vi "Status Created Events.vi"(7 "jettl in":refnum<class "jettl.lvclass">, 10 "Queue Mailbox":refnum<data-value>) -> (0 "Created Event Count":i32, 1 "Created Event Aliases":string[](array[string]), 2 "Created Event Exist?":bool, 5 "jettl out":refnum<class "jettl.lvclass">)   [LabVIEW 2021, in "jettl.lvlib" / "Addresses.lvlib"]
uses:
  Addresses.lvlib
  Addresses/Addresses.lvclass
  jettl/jettl.lvclass
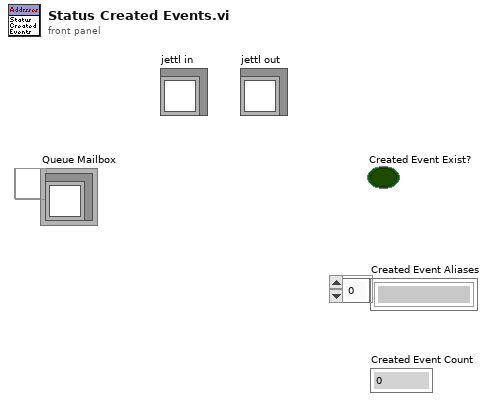
[diagram p1: front panel]
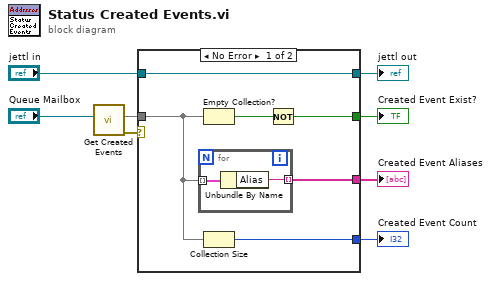
[diagram p0: block diagram]
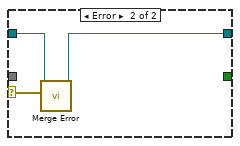
[diagram p2: hidden frame]
diagram:
  n1 = call "Get Created Events.vi"("Queue Mailbox"="Queue Mailbox") -> ("error out"=w3:errorcluster, "Created Events"=w2:map{string, refnum<data-value>})  [unwired: 9 in]
  n2 = case shown="No Error" w3 {
    selector: w3 -> [_ w17]
    tunnel: [w13 _] -> w8
    tunnel: [w12 _] -> w7
    tunnel: [w11 _] -> w6
    tunnel: w2 -> [w10 _]
    tunnel: [w9 w18] -> w5
    tunnel: "jettl in" -> [w9 w19]
    frame No Error {
      n3 = for {
        tunnel: [w15] -> w12 mode=indexing
        tunnel: w10 -> [w16] mode=indexing
        n4 = Unbundle By Name(w16) -> ("Alias"=w15:string)
      }
      n5 = Empty Collection?(1:w10) -> (0:w14:bool)
      n6 = Collection Size(1:w10) -> (0:w11:i32)
      n7 = Not(x=w14) -> (.not. x?=w13:bool)
    }
    frame Error {
      n8 = call-dynamic "Merge Error.vi"("Error"=w17, "Merge Error in"=w19) -> ("Merge Error out"=w18:refnum<class "jettl.lvclass">)  [unwired: 9 in]
    }
  }
  "Created Event Aliases" <- w7
  "Created Event Exist?" <- w8
  "Created Event Count" <- w6
  "jettl out" <- w5
